vi "FTW-Router-Worker.vi"(0 "Backend Handler":refnum<user-event>, 2 "RouterID":i64 format="%016x") -> ()   [LabVIEW 2013, in "FTW-Router.lvclass"]
uses:
  FTW-Router.lvclass
  message/FTW-Message.lvclass
  error/FTW-ERR-ThrowGenericError.vi
  error/FTW-ERR-ThrowError.vi
  error/FTW-ERR-CallChain.vi
  string/FTW-STR-ReplaceWhitespace.vi
  socket/FTW-Socket.lvclass
panel:
  out "recv err":errorcluster
  out "Iteration":i32
  out "Incoming Messages":i32
  # "Inputs"
  # "Debug"
  # "Outputs"
  # "This asynchronous worker has no outputs"
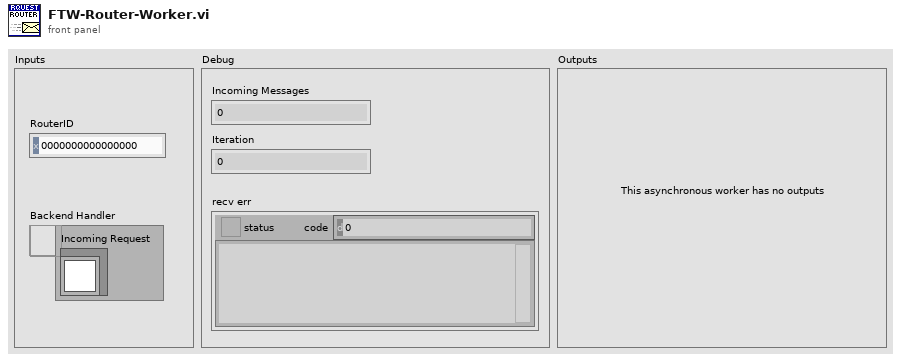
[diagram p1: front panel]
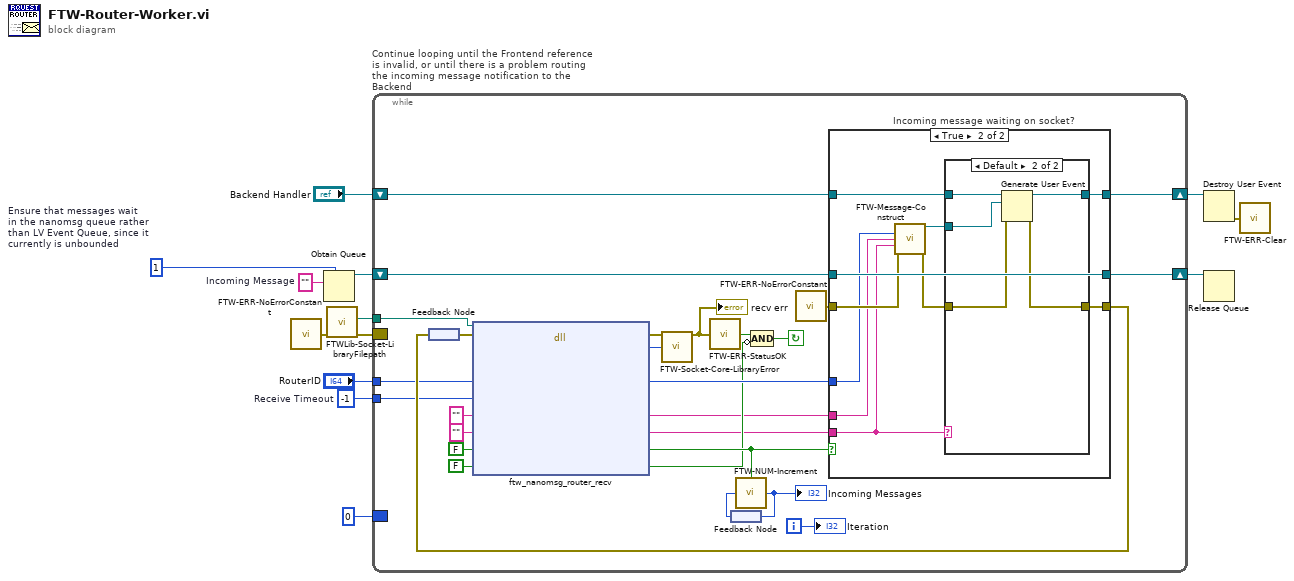
[diagram p0: block diagram]
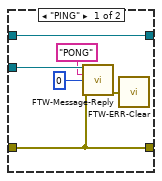
[diagram p3: hidden frame]
diagram:
  w4 = -1  # Receive Timeout
  w8 = ""  # Incoming Message
  w9 = 1  # Ensure that messages wait in the nanomsg queue rather than LV Event Queue, since it currently is unbounded
  n1 = call "FTW-ERR-NoErrorConstant.vi"() -> ("no error"=w2:errorcluster)
  n2 = Obtain Queue(max queue size (-1, unlimited)=w9, element data type=w8) -> (queue out=w10:refnum<queue>)  [unwired: 3 in, 2 out]
  n3 = call "FTWLib-Socket-LibraryFilepath.vi"("error in"=w2) -> ("error out"=w1:errorcluster, "Library Filepath"=w3:path)  [unwired: 8 in, 1 out]
  n4 = while "Continue looping until the Frontend reference is invalid, or until there is a problem routing the incoming message notification to the Backend" {
    border: w1 -> [_]
    shift-right: [w38] -> w12
    shift-left: "Backend Handler" -> [w40]
    border: 0 ("Messages Handled") -> [_]
    tunnel: "RouterID" -> [w32]
    shift-right: [w31] -> w6
    shift-left: w10 -> [w35]
    tunnel: w4 -> [w27]
    tunnel: w3 -> [w25]
    i -> [w36]
    stop <- w22 continue-if-true
    n5 = feedback #1() -> (w24:errorcluster)
    n6 = dll-call lib="?" fn="ftw_nanomsg_router_recv"(path in=w25, error in=w24, "RouterID"=w32, "Timeout"=w27, "Backtrace"="", "Incoming Request"="", "Message Received?"=FALSE, "Shutdown?"=FALSE) -> (error out=w29:errorcluster, "Return Value"=w30:i64, "RouterID"=w26:i64, "Backtrace"=w15:string, "Incoming Request"=w14:string, "Message Received?"=w17:bool, "Shutdown?"=w16:bool)  [unwired: 4 in, 1 out]
    n7 = call "FTW-Socket-Core-LibraryError.vi"("error in"=w29, "Return Value"=w30) -> ("error out"=w28:errorcluster)  [unwired: 13 in]
    "recv err" <- w28
    n8 = call "FTW-ERR-StatusOK.vi"("error to check"=w28) -> ("Status OK?"=w23:bool)
    n9 = feedback #2() -> (w33:i32)
    n10 = call "FTW-NUM-Increment.vi"("Initial Value"=w33, "Increment?"=w17) -> ("Final Value"=w34:i32)
    "Incoming Messages" <- w34
    n11 = feedback-in #2(w34) -> ()
    n12 = Compound Arithmetic op=AND(w23, invert w16) -> (w22:bool)
    n13 = call "FTW-ERR-NoErrorConstant.vi"() -> ("no error"=w37:errorcluster)
    n14 = case "Incoming message waiting on socket?" shown="True" w17 {
      tunnel: w40 -> [w43 w53]
      tunnel: [w42 w51] -> w39
      tunnel: [w43 w52] -> w38
      tunnel: w37 -> [w42 w49]
      tunnel: w35 -> [w41 w50]
      tunnel: [w41 w50] -> w31
      tunnel: w15 -> [_ w45]
      tunnel: w14 -> [_ w44]
      tunnel: w26 -> [_ w46]
      frame False {
      }
      frame True {
        n15 = call "FTW-Message-Construct.vi"("RouterID"=w46, "Backtrace"=w45, "Incoming Message"=w44, "error in"=w49) -> ("FTW Incoming Message"=w48:refnum<class "FTW-Message.lvclass">, "error out"=w47:errorcluster)  [unwired: 10 in]
        n16 = case shown="Default" w44 {
          tunnel: w53 -> [w59 w64]
          tunnel: [w59 w63] -> w52
          tunnel: [w57 w62] -> w51
          tunnel: w48 -> [w58 w61]
          tunnel: w47 -> [w57 w60]
          frame "PING" {
            n17 = call "FTW-Message-Reply.vi"("FTW Incoming Message"=w58, "Response"="PONG", "Send Timeout"=0, "error in"=w57) -> ("error out"=w54:errorcluster)  [unwired: 10 in, 1 out]
            n18 = call "FTW-ERR-Clear.vi"("error to snuff"=w54) -> ()  [unwired: 1 out]
          }
          frame Default {
            n19 = Generate User Event(user event=w64, event data cluster=w61, error in=w60) -> (user event out=w63:refnum<user-event>, error out=w62:errorcluster)  [unwired: 1 in]
          }
        }
      }
    }
    n20 = feedback-in #1(w39) -> ()
    "Iteration" <- w36
  }
  n21 = Destroy User Event(user event=w12) -> (error out=w7:errorcluster)  [unwired: 1 in]
  n22 = Release Queue(queue=w6) -> ()  [unwired: 2 in, 3 out]
  n23 = call "FTW-ERR-Clear.vi"("error to snuff"=w7) -> ()  [unwired: 1 out]
